vi "Calculate Pulse Width from Waveform.vi"(11 "Samples":waveform(dbl)={"t0"=timestamp(0 s since 1904-01-01), "dt"=0.0, "Y"=[]}) -> (3 "Pulse Width":dbl)   [LabVIEW 2010]
uses:
  <vilib>/measure/mascope.llb/Pulse Measurements 1 chan.vi
  <vilib>/measure/NI_MAPro.lvlib
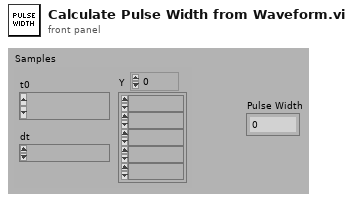
[diagram p1: front panel]
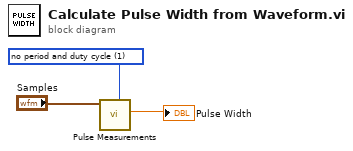
[diagram p0: block diagram]
diagram:
  w2 = u16 1 items=["all", "no period and duty cycle"] ("export mode")
  n1 = call-poly <vilib>:"Pulse Measurements.vi"("export mode"=w2, "signal in"="Samples") -> ("pulse duration"=→"Pulse Width":dbl)  [unwired: 5 in, 4 out]
